vi "sysexecsubvi.vi"   [LabVIEW 2014]
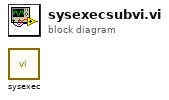
[diagram p0: block diagram]
diagram:
  n1 = call "sysexec.vi"() -> ()  [unwired: 12 in]
